vi "erstes.vi"() -> ()   [LabVIEW 2010]
uses:
  <vilib>/Utility/file.llb/Write To Spreadsheet File (DBL).vi
  <vilib>/Analysis/NI_AALBase.lvlib
panel:
  in  "Stop 5":dbl format="%.2f"
  in  "Stop 4":dbl format="%.2f"
  in  "Stop 3":dbl format="%.2f"
  in  "Start 5":dbl format="%.2f"
  in  "Start 4":dbl format="%.2f"
  in  "Start 3":dbl format="%.2f"
  out "Numeric 2":dbl format="%.2f"
  in  "Step 2":dbl format="%.2f"
  in  "Stop 2":dbl format="%.2f"
  in  "Start 2":dbl format="%.2f"
  out "data":string
  out "Numeric":dbl format="%.2f"
  out "XY Graph 2":cluster{dbl[], dbl[]}(graph)
  out "XY Graph":cluster{dbl[], dbl[]}(graph)
  in  "Path":path
  out "error out 2":errorcluster
  in  "Wait/s":dbl format="%.2f"
  in  "Step":dbl format="%.2f"
  in  "error in (no error)":errorcluster
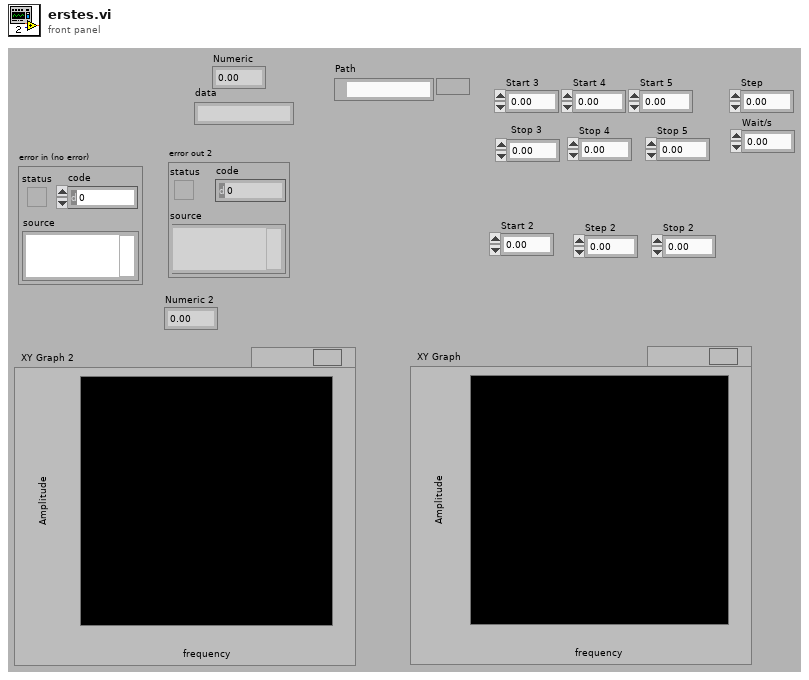
[diagram p1: front panel]
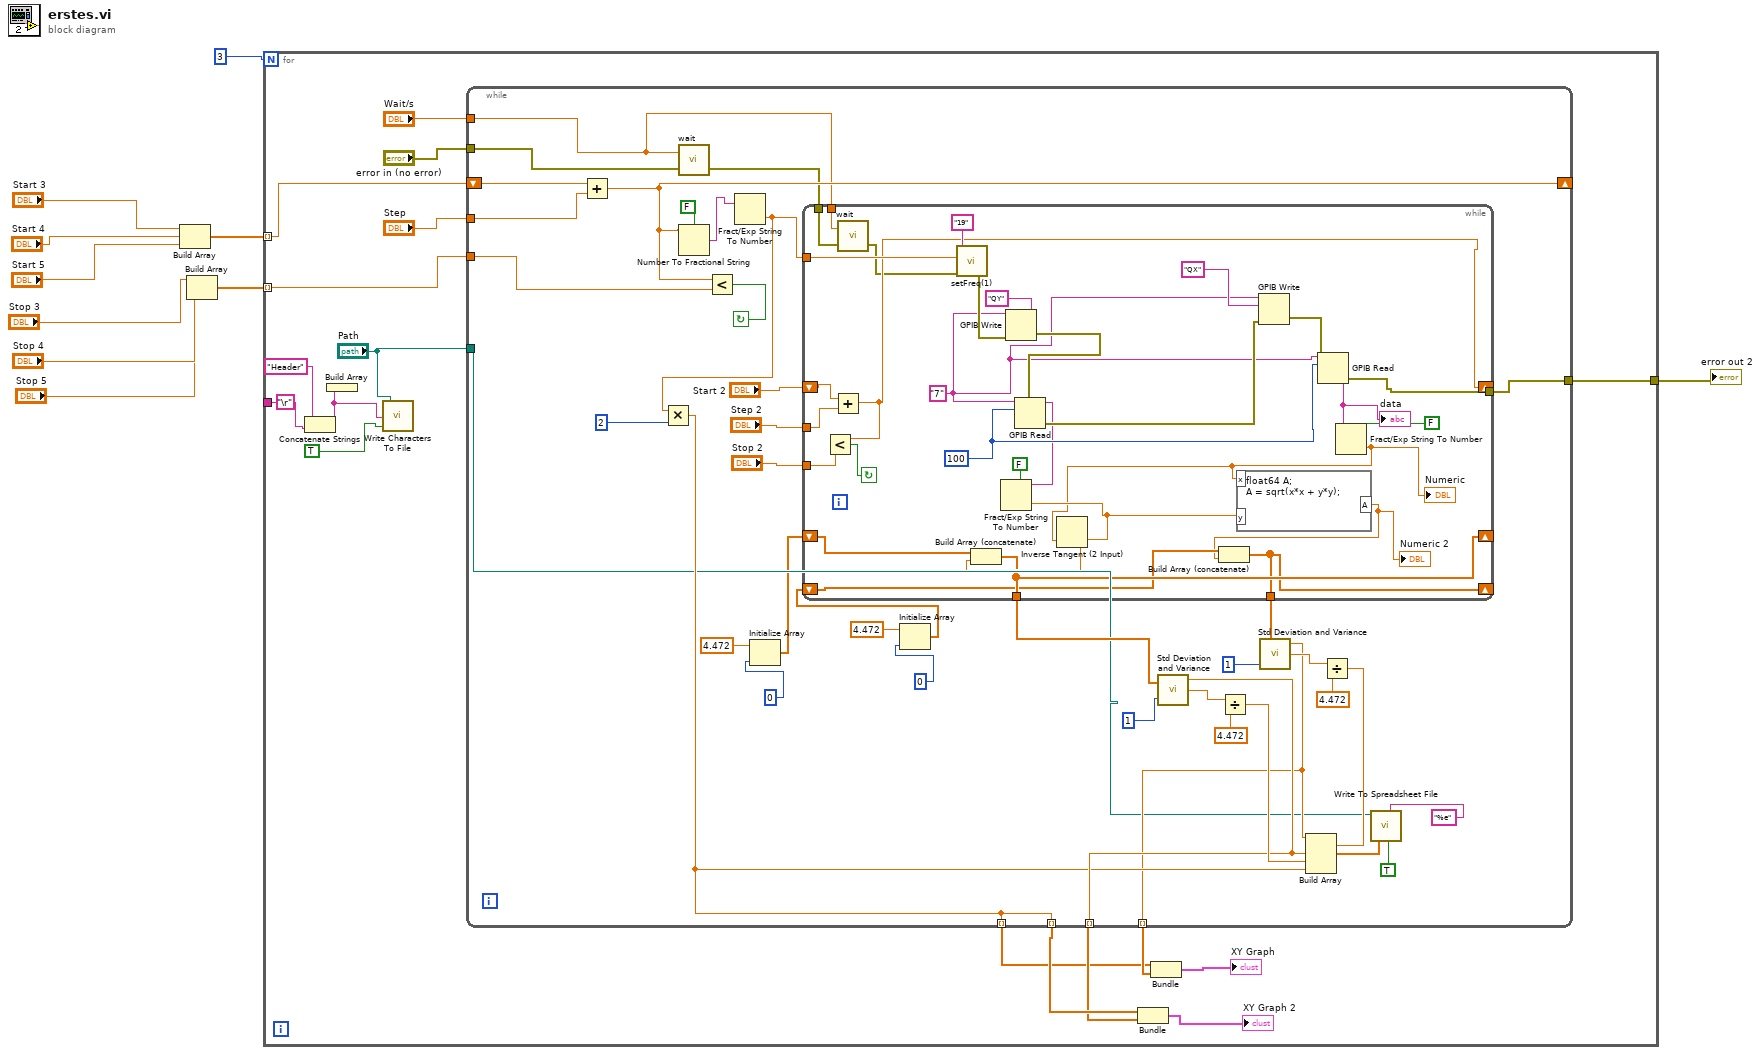
[diagram p0: block diagram]
diagram:
  n1 = Build Array("Start 3", "Start 4", "Start 5") -> (w2:dbl[])
  n2 = Build Array("Stop 3", "Stop 4", "Stop 5") -> (w1:dbl[])
  n3 = for {
    N: 3 -> [_]
    tunnel: "\r" -> [w24]
    tunnel: [w14] -> w10
    tunnel: w2 -> [w13] mode=indexing
    tunnel: w1 -> [w12] mode=indexing
    n4 = Concatenate Strings("Header", w24) -> (w22:string)
    n5 = Build Array(w22) -> ()  [unwired: 1 out]
    n6 = call <vilib>:"Write Characters To File.vi"("append to file? (new file:F)"=TRUE, "character string"=w22, "file path (dialog if empty)"="Path") -> ()  [unwired: 2 in, 1 out]
    n7 = while {
      tunnel: "error in (no error)" -> [w61]
      shift-right: [w62] -> _
      shift-left: w13 -> [w65]
      tunnel: "Step" -> [w67]
      tunnel: w12 -> [w66]
      tunnel: "Wait/s" -> [w38]
      tunnel: "Path" -> [w35]
      tunnel: [w56] -> w14
      tunnel: [w42] -> w18 mode=indexing
      tunnel: [w43] -> w17 mode=indexing
      tunnel: [w42] -> w15 mode=indexing
      tunnel: [w40] -> w16 mode=indexing
      stop <- w64 continue-if-true
      n8 = Add(x=w65, y=w67) -> (x+y=w62:dbl)
      n9 = call "wait.vi"("error in"=w61, "Wartezeit in Sek"=w38) -> ("error out"=w60:errorcluster)  [unwired: 1 in]
      n10 = Number To Fractional String(use system decimal point (T)=FALSE, number=w62) -> (F-format string=w59:string)  [unwired: 2 in]
      n11 = Less?(x=w62, y=w66) -> (x < y?=w64:bool)
      n12 = Fract/Exp String To Number(string=w59) -> (number=w52:dbl)  [unwired: 3 in, 1 out]
      n13 = Multiply(x=w52, y=2) -> (x*y=w42:dbl)
      n14 = Initialize Array(4.472, 0) -> (w32:dbl[])
      n15 = Initialize Array(4.472, 0) -> (w29:dbl[])
      n16 = while {
        tunnel: w60 -> [w76]
        tunnel: w52 -> [w94]
        tunnel: [w89] -> w56
        tunnel: "Step 2" -> [w82]
        tunnel: "Stop 2" -> [w81]
        tunnel: [w70] -> w51
        tunnel: [w72] -> w45
        shift-right: [w78] -> _
        shift-left: "Start 2" -> [w79]
        tunnel: w38 -> [w77]
        shift-right: [w72] -> _
        shift-left: w32 -> [w73]
        shift-right: [w70] -> _
        shift-left: w29 -> [w71]
        stop <- w80 continue-if-true
        w88 = 100
        w90 = "7"
        n17 = Add(x=w79, y=w82) -> (x+y=w78:dbl)
        n18 = Less?(x=w78, y=w81) -> (x < y?=w80:bool)
        n19 = call "wait.vi"("error in"=w76, "Wartezeit in Sek"=w77) -> ("error out"=w75:errorcluster)  [unwired: 1 in]
        n20 = call "setFreq(1).vi"("error in"=w75, "Frequenz in Hz"=w94, "address string"="19") -> ("error out"=w95:errorcluster)  [unwired: 3 in]
        n21 = GPIB Write(0:w90, 1:"QY", 3:w95) -> (6:w96:errorcluster)  [unwired: 2 in, 1 out]
        n22 = GPIB Read(0:w90, 1:w88, 3:w96) -> (5:w86:string, 7:w92:errorcluster)  [unwired: 2 in, 1 out]
        n23 = Fract/Exp String To Number(use system decimal point (T)=FALSE, string=w86) -> (number=w87:dbl)  [unwired: 2 in, 1 out]
        n24 = GPIB Write(0:w90, 1:"QX", 3:w92) -> (6:w91:errorcluster)  [unwired: 2 in, 1 out]
        n25 = GPIB Read(0:w90, 1:w88, 3:w91) -> (5:w84:string, 7:w89:errorcluster)  [unwired: 2 in, 1 out]
        "data" <- w84
        n26 = Fract/Exp String To Number(use system decimal point (T)=FALSE, string=w84) -> (number=w85:dbl)  [unwired: 2 in, 1 out]
        "Numeric" <- w85
        n27 = Inverse Tangent (2 Input)(1:w85, 2:w87) -> (0:w74:dbl)
        n28 = Build Array (concatenate)(w73, w74) -> (w72:dbl[])
        n29 = formula code="float64 A;\nA = sqrt(x*x + y*y);"("x"=w85, "y"=w87) -> ("A"=w69:dbl)
        "Numeric 2" <- w69
        n30 = Build Array (concatenate)(w71, w69) -> (w70:dbl[])
      }
      n31 = call <vilib>:"Std Deviation and Variance.vi"("X"=w45, "Weighting (Sample)"=1) -> ("mean"=w43:dbl, "standard deviation"=w47:dbl)  [unwired: 1 out]
      n32 = Divide(x=w47, y=4.472) -> (x/y=w44:dbl)
      n33 = call <vilib>:"Std Deviation and Variance.vi"("X"=w51, "Weighting (Sample)"=1) -> ("mean"=w40:dbl, "standard deviation"=w50:dbl)  [unwired: 1 out]
      n34 = Divide(x=w50, y=4.472) -> (x/y=w48:dbl)
      n35 = Build Array(w40, w48, w43, w44, w42) -> (w41:dbl[])
      n36 = call-poly <vilib>:"Write To Spreadsheet File.vi"("format (%.3f)"="%e", "append to file? (new file:F)"=TRUE, "1D data"=w41, "file path (dialog if empty)"=w35) -> ()  [unwired: 4 in, 1 out]
    }
    n37 = Bundle(w18, w17) -> (→"XY Graph 2":cluster{dbl[], dbl[]})  [unwired: 1 in]
    n38 = Bundle(w15, w16) -> (→"XY Graph":cluster{dbl[], dbl[]})  [unwired: 1 in]
  }
  "error out 2" <- w10
